vi "3D Waterfall Graph.vi"() -> ()   [LabVIEW 2020]
doc: "This VI shows how to use the 3D Waterfall Plot."
uses:
  <vilib>/Math Plots/3D Math Plots/3D Waterfall/3D Waterfall XCtrl/3D Waterfall.xctl
  <vilib>/Math Plots/3D Math Plots/3D Waterfall/3D Waterfall Datatype/Public/Plot Helper (Vector).vi
  <vilib>/Math Plots/3D Math Plots/3D Waterfall/3D Waterfall Datatype/3D Waterfall Datatype.lvclass
panel:
  out "3D Waterfall":refnum<class "3D Plot Datatype.lvclass">[](xcontrol)
  # "Overview: Demonstrates the Waterfall indicator from the Graph > 3D Graph palette.\nRequirements: LabVIEW Full Development System\nInstructions:\nRun the VI."
  # "Try the following operations on the graph:\n\n1. Click and drag the mouse within the graph to change the view direction.\n2. Press the Shift key and drag the mouse up to zoom in.\n3. Press the Shift key and drag the mouse down to zoom out.\n4. Right-click the graph and choose 3D Plot Properties to configure various properties related to the graph's appearance.\n5. Right-click the graph and select Export Image >Export to File."
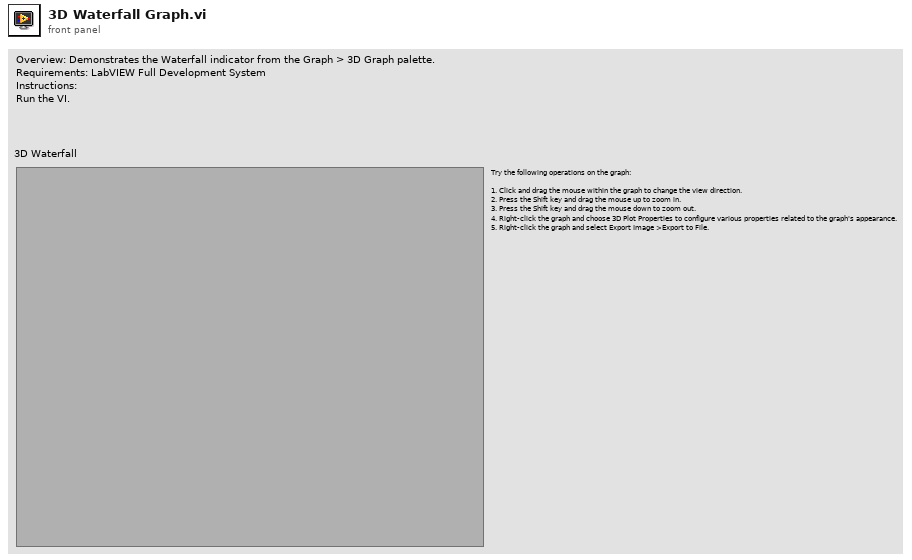
[diagram p1: front panel]
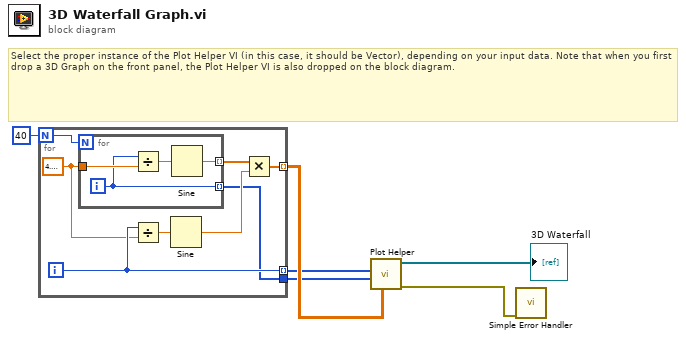
[diagram p0: block diagram]
diagram:
  # "Select the proper instance of the Plot Helper VI (in this case, it should be Vector), depending on your input data. Note that when you first drop a 3D Graph on the front panel, the Plot Helper VI is also dropped on the block diagram."
  n1 = for {
    N: 40 ("X input length") -> [w9]
    tunnel: [w11] -> w4 mode=indexing
    tunnel: [w10] -> w3 mode=indexing
    tunnel: [w7] -> w2
    i -> [w10]
    w8 = sgl 4.2 ("y")
    n2 = for {
      N: w9 -> [_]
      tunnel: [w17] -> w13 mode=indexing
      tunnel: w8 -> [w16]
      tunnel: [w15] -> w7 mode=indexing
      i -> [w15]
      n3 = Divide(x=w15, y=w16) -> (x/y=w18:sgl)
      n4 = Sine(x=w18) -> (sin(x)=w17:sgl)
    }
    n5 = Divide(x=w10, y=w8) -> (x/y=w14:sgl)
    n6 = Sine(x=w14) -> (sin(x)=w12:sgl)
    n7 = Multiply(x=w13, y=w12) -> (x*y=w11:sgl[])
  }
  n8 = call-poly <vilib>:"Plot Helper.vi"("z matrix"=w4, "y vector"=w2, "x vector"=w3) -> ("error out"=w1:errorcluster, "3D Plot lvclass Array out"=→"3D Waterfall":refnum<class "3D Plot Datatype.lvclass">[])  [unwired: 3 in, 4 out]
  n9 = call <vilib>:"Simple Error Handler.vi"("error in (no error)"=w1) -> ()  [unwired: 4 in, 5 out]
